vi "TEST - Get TDEnum from TD.vi"(8 "error in (no error)":errorcluster) -> (0 "error out":errorcluster, 2 "pass":bool)   [LabVIEW 2020]
uses:
  source/library/Type Descriptor.ctl
  source/library/Type Descriptor Enumeration.ctl
  source/library/openg_variant.lvlib
panel:
  out "Failures":T3(array[cluster]) {"result"."Type Descriptor Enumeration" format="%.0x"; "exected result"."Type Descriptor Enumeration" format="%.0x"}
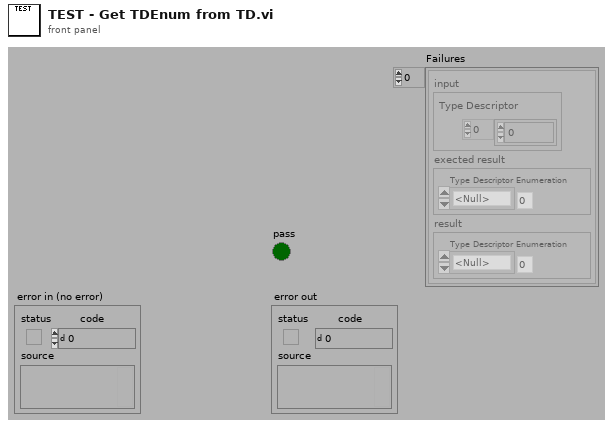
[diagram p1: front panel]
types:
  T1 = typedef "openg_variant.lvlib/Type Descriptor.ctl" = i16[]
  T2 = typedef "openg_variant.lvlib/Type Descriptor Enumeration.ctl" = enum8{"<Null>", "I8", "I16", "I32", "I64", "U8", "U16", "U32", "U64", "SGL", "DBL", "EXT", "CSG", "CDB", "CXT", "0x0F", "0x10", "0x11", "0x12", "0x13", "0x14", "Enum U8", "Enum U16", "Enum U32", "Enum U64", "SGL PQ", "DBL PQ", "EXT PQ", "CSG PQ", "CDB PQ", "CXT PQ", "0x1F", "0x20", "Boolean", "0x22", "0x23", "0x24", "0x25", "0x26", "0x27", "0x28", "0x29", "0x2A", "0x2B", "0x2C", "0x2D", "0x2E", "0x2F", "String", "0x31", "Path", "Pict", "0x34", "0x35", "0x36", "DAQ", "0x38", "0x39", "0x3A", "0x3B", "0x3C", "0x3D", "0x3E", "0x3F", "Array", "0x41", "0x42", "0x43", "0x44", "0x45", "0x46", "0x47", "0x48", "0x49", "0x4A", "0x4B", "0x4C", "0x4D", "0x4E", "0x4F", "Cluster", "0x51", "0x52", "Variant", "Waveform", "0x55", "0x56", "0x57", "0x58", "0x59", "0x5A", "0x5B", "0x5C", "0x5D", "0x5E", "Fixed Point", "0x60", "0x61", "0x62", "0x63", "0x64", "0x65", "0x66", "0x67", "0x68", "0x69", "0x6A", "0x6B", "0x6C", "0x6D", "0x6E", "0x6F", "Refnum", "0x71", "0x72", "Set Collection", "Map Collection"}
  T3 = cluster{"input":cluster{"Type Descriptor":T1}, "exected result":cluster{"Type Descriptor Enumeration":T2}, "result":cluster{"Type Descriptor Enumeration":T2}}[]
  T4 = cluster{"input":cluster{"Type Descriptor":T1}, "exected result":cluster{"Type Descriptor Enumeration":T2}, "result":cluster{"Type Descriptor Enumeration":T2}}
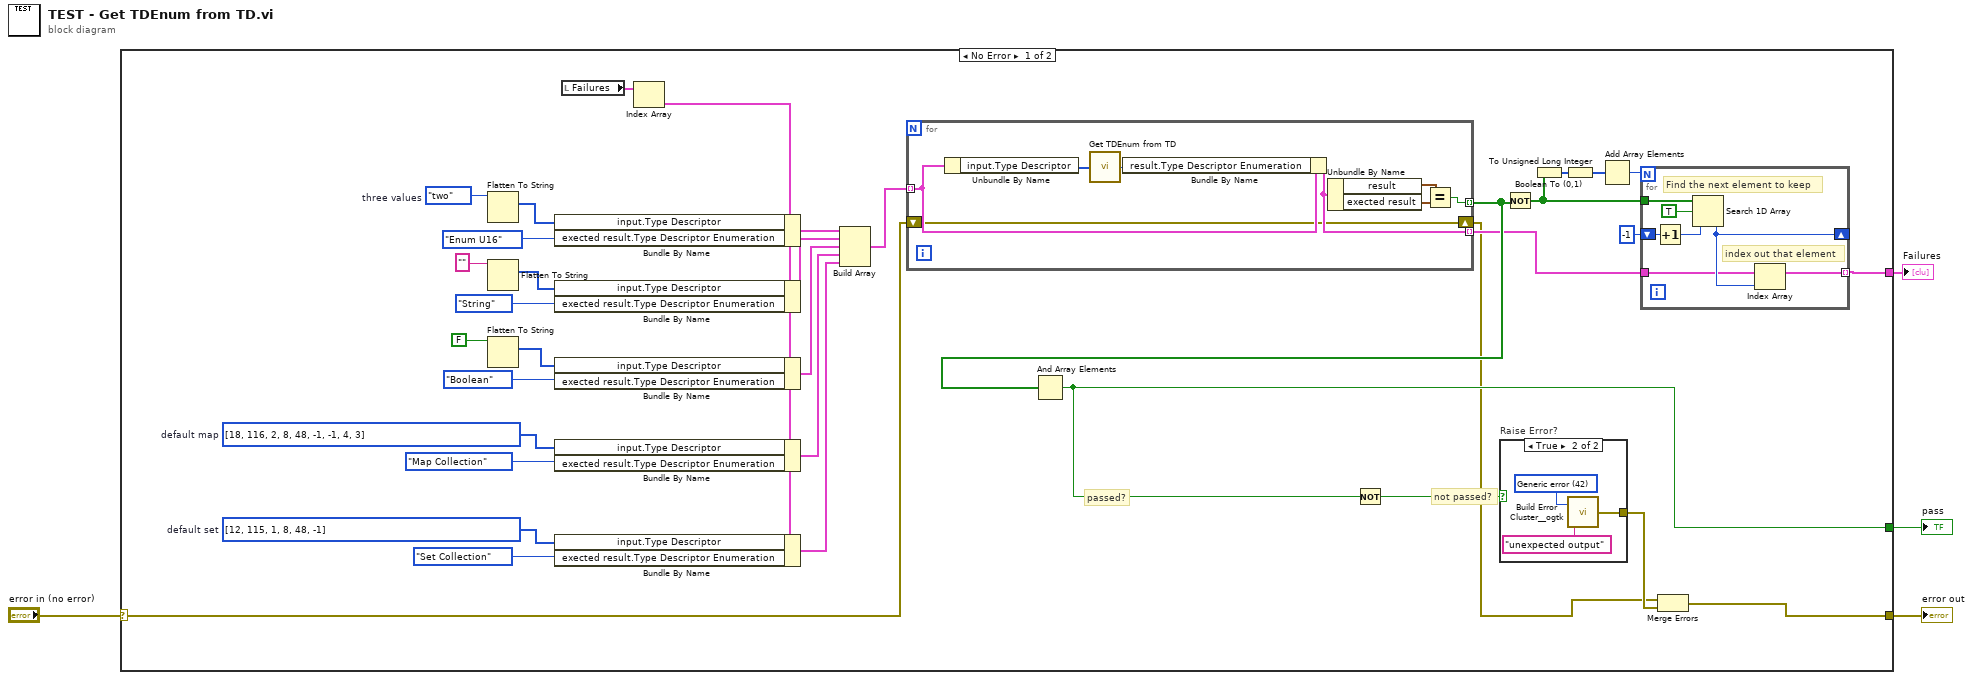
[diagram p0: block diagram]
diagram:
  n1 = case shown="No Error" "error in (no error)" {
    selector: "error in (no error)" -> [w25 w58]
    tunnel: [w36 _] -> w4
    tunnel: [w39 w58] -> w2
    tunnel: [w28 _] -> w1
    frame No Error {
      w8 = i16[] [12, 115, 1, 8, 48, -1]  # default set
      w10 = i16[] [18, 116, 2, 8, 48, -1, -1, 4, 3]  # default map
      w18 = enum16{"one", "two", "three"}."two"  # three values
      # "not passed?"
      # "passed?"
      n2 = Flatten To String(anything=w18) -> (type string=w17:i16[])  [unwired: 3 in, 2 out]
      n3 = Flatten To String(anything="") -> (type string=w13:i16[])  [unwired: 3 in, 2 out]
      n4 = Flatten To String(anything=FALSE) -> (type string=w14:i16[])  [unwired: 3 in, 2 out]
      n5 = local read "Failures"() -> (w23:T3)
      n6 = Index Array(array=w23) -> (element=w6:T4)  [unwired: 1 in]
      n7 = Bundle By Name(cluster=w6, "input.Type Descriptor"=w17, "exected result.Type Descriptor Enumeration"=Type_Descriptor_Enumeration."Enum U16") -> (w27:T4)
      n8 = Bundle By Name(cluster=w6, "input.Type Descriptor"=w13, "exected result.Type Descriptor Enumeration"=Type_Descriptor_Enumeration."String") -> (w20:T4)
      n9 = Bundle By Name(cluster=w6, "input.Type Descriptor"=w14, "exected result.Type Descriptor Enumeration"=Type_Descriptor_Enumeration."Boolean") -> (w19:T4)
      n10 = Bundle By Name(cluster=w6, "input.Type Descriptor"=w10, "exected result.Type Descriptor Enumeration"=Type_Descriptor_Enumeration."Map Collection") -> (w9:T4)
      n11 = Bundle By Name(cluster=w6, "input.Type Descriptor"=w8, "exected result.Type Descriptor Enumeration"=Type_Descriptor_Enumeration."Set Collection") -> (w5:T4)
      n12 = Build Array(w27, w20, w19, w9, w5) -> (w26:T3)
      n13 = for {
        tunnel: w26 -> [w53] mode=indexing
        tunnel: [w54] -> w30 mode=indexing
        tunnel: [w52] -> w29 mode=indexing
        shift-right: [w47] -> w24
        shift-left: w25 -> [w47]
        n14 = Unbundle By Name(w53) -> ("input.Type Descriptor"=w49:T1)
        n15 = call "Get TDEnum from TD.vi"("Type Descriptor"=w49) -> ("Type Descriptor Enumeration"=w48:T2)  [unwired: 4 in]
        n16 = Bundle By Name(cluster=w53, "result.Type Descriptor Enumeration"=w48) -> (w52:T4)
        n17 = Unbundle By Name(w52) -> ("result"=w51:cluster{"Type Descriptor Enumeration":T2}, "exected result"=w50:cluster{"Type Descriptor Enumeration":T2})
        n18 = Equal?(x=w51, y=w50) -> (x = y?=w54:bool)
      }
      n19 = And Array Elements(Boolean array=w30) -> (logical AND=w36:bool)
      n20 = Not(x=w36) -> (.not. x?=w37:bool)
      n21 = case "Raise Error?" shown="True" w37 {
        tunnel: [_ w55] -> w38
        frame False {
        }
        frame True {
          w56 = 42 items=["No error", "Argument error", "Memory is full", "Out of zone", "End of file", "File already open", "Generic file I/O error", "File not found", "File permission error", "Disk is full", "Duplicate path", "Too many files open", "System feature not enabled", "Resource file not found", "Cannot add resource", "Resource not found", "Image not found", "Image memory error", "Pen does not exist", "Config type invalid", "Config token not found", "Config parse error", "Config memory error", "Bad external code format", "Bad external code offset", "External code not present", "Null window", "Destroy window error", "Null menu", "Print aborted", "Bad print record", "Print driver error", "Windows error during printing", "Memory error during printing", "Print dialog error", "Generic print error", "Invalid device refnum", "Device not found", "Device parameter error", "Device unit error", "Cannot open device", "Device call aborted", "Generic error", "Cancelled by user", "Object ID too low", "Object ID too high", "Object not in heap", "Unknown heap", "Unknown object (invalid DefProc)", "Unknown object (DefProc not in table)", "Message out of range", "Invalid (null) method", "Unknown message", "Manager call not supported", "Bad address", "Network operation in progress", "Network operation timed out", "Connection is busy", "Network attribute not supported", "Network error", "Address in use", "System out of memory", "Connection aborted", "Connection refused", "Not connected", "Already connected", "Connection closed", "Initialization error (interapplication manager)", "Bad occurrence", "Wait on unbound occurrence handler", "Occurrence queue overflow", "Datalog type conflict", "Unused", "Unrecognized type (interapplication manager)", "Memory corrupt", "Failed to make temporary DLL", "Old CIN version", "Drag socket not found", "Failed to load drop-object", "Failed to register OLE object", "Failed to release OLE object", "Format specifier type mismatch", "Unknown format specifier", "Too few format specifiers", "Too many format specifiers", "Scan failed", "Newer CIN version", "Error converting to variant", "Runtime menu error", "Password tampered", "Variant attribute not found", "Incompatible variant data type", "Event data is not available", "Event Store is not present", "Occurrence is not found", "Event Queue is not created", "Event info is not available", "Refnum passed is NULL", "Error retrieving Class GUID", "Error retrieving CoClass GUID", "Error retrieving TypeLib GUID.", "Bad built application magic bytes.", "Specific driver is different from the specific driver associated with the Logical Name.", "There is no session opened to the class driver.", "Max Error", "MAX - Error with config objects", "MAX - Error loading configuration", "MAX - Group not supported"]
          n22 = call <userlib>:"Build Error Cluster__ogtk.vi"("String to Prepend to source (\"\")"="unexpected output" ("String to Prepend to source (\"\")"), "code"=w56) -> ("error out"=w55:errorcluster)
        }
      }
      n23 = Not(x=w30) -> (.not. x?=w32:bool[])
      n24 = Boolean To (0,1)(Boolean=w32) -> (0, 1=w33:i16[])
      n25 = To Unsigned Long Integer(number=w33) -> (unsigned 32bit integer=w31:u32[])
      n26 = Add Array Elements(numeric array=w31) -> (sum=w34:u32)
      n27 = for {
        N: w34 -> [_]
        tunnel: w29 -> [w42]
        tunnel: w32 -> [w46]
        shift-right: [w43] -> _
        shift-left: -1 ("start index (0)") -> [w44]
        tunnel: [w41] -> w28 mode=indexing
        # "index out that element"
        # "Find the next element to keep"
        n28 = Increment(x=w44) -> (x+1=w40:i32)
        n29 = Search 1D Array(1D array=w46, element=TRUE, start index (0)=w40) -> (index of element=w43:i32)
        n30 = Index Array(array=w42, index=w43) -> (element=w41:T4)
      }
      n31 = Merge Errors(w24, w38) -> (w39:errorcluster)
    }
    frame Error {
    }
  }
  "pass" <- w4
  "error out" <- w2
  "Failures" <- w1
